vi "Bin to BDC(4-разрядное число).vi"(3 "B":T2) -> (0 "D1":T1, 1 "D0":T1)   [LabVIEW 2013]
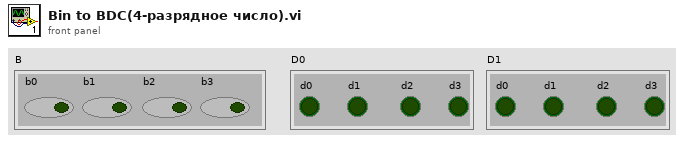
[diagram p1: front panel]
types:
  T1 = cluster{"d0":bool, "d1":bool, "d2":bool, "d3":bool}
  T2 = cluster{"b0":bool, "b1":bool, "b2":bool, "b3":bool}
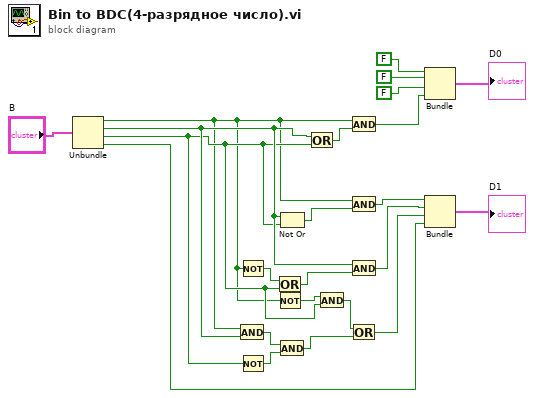
[diagram p0: block diagram]
diagram:
  n1 = Unbundle("B") -> ("b0"=w1:bool, "b1"=w8:bool, "b2"=w2:bool, "b3"=w6:bool)
  n2 = And(x=w1, y=w8) -> (x .and. y?=w9:bool)
  n3 = Not(x=w1) -> (.not. x?=w3:bool)
  n4 = Not(x=w2) -> (.not. x?=w7:bool)
  n5 = Or(x=w3, y=w2) -> (x .or. y?=w12:bool)
  n6 = Not(x=w1) -> (.not. x?=w4:bool)
  n7 = Not Or(1:w2, 2:w8) -> (0:w15:bool)
  n8 = And(x=w9, y=w7) -> (x .and. y?=w10:bool)
  n9 = Or(x=w8, y=w2) -> (x .or. y?=w17:bool)
  n10 = And(x=w4, y=w2) -> (x .and. y?=w5:bool)
  n11 = And(x=w1, y=w17) -> (x .and. y?=w16:bool)
  n12 = And(x=w1, y=w15) -> (x .and. y?=w14:bool)
  n13 = And(x=w8, y=w12) -> (x .and. y?=w13:bool)
  n14 = Or(x=w5, y=w10) -> (x .or. y?=w11:bool)
  n15 = Bundle(FALSE, FALSE, FALSE, w16) -> (→"D0":cluster{bool, bool, bool, bool})  [unwired: 1 in]
  n16 = Bundle(w14, w13, w11, "b3"=w6) -> (→"D1":cluster{bool, bool, bool, "b3":bool})  [unwired: 1 in]
